vi "AssetInterface_Write Process Name.vi"(10 "Process Name":string, 11 "Load in":refnum<class "Load.lvclass">) -> (3 "Load out":refnum<class "Load.lvclass">)   [LabVIEW 2015, in "Load.lvclass"]
uses:
  Load.lvclass
  Load.lvclass/Load.ctl
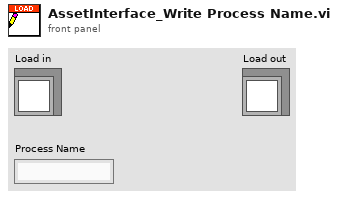
[diagram p1: front panel]
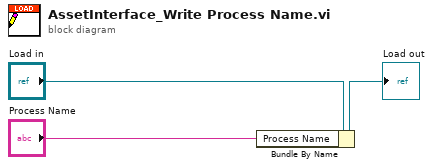
[diagram p0: block diagram]
diagram:
  n1 = Bundle By Name(cluster="Load in", "Process Name"="Process Name") -> (→"Load out":refnum<class "Load.lvclass">)
